vi "Configure.vi"(8 "error in (no error)":errorcluster, 11 "Hardware Refs In":T1={"IP Address"="Simulator", "Handle"=0, "Refresh Time (ms)"=0.0}) -> (0 "error out":errorcluster, 3 "Hardware Refs Out":T1={"IP Address"="Simulator", "Handle"=0, "Refresh Time (ms)"=0.0})   [LabVIEW 2013, in "Capacitive.lvlib"]
uses:
  Capacitive.lvlib
  Hardware Configuration.ctl
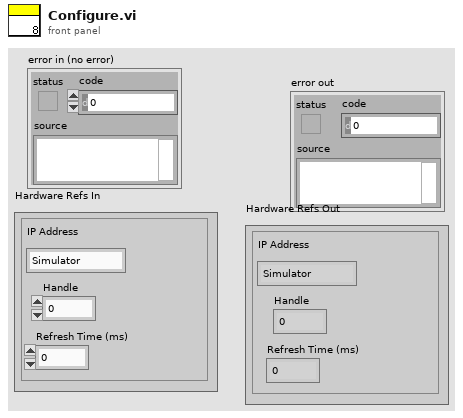
[diagram p1: front panel]
types:
  T1 = typedef "Capacitive.lvlib/Hardware Configuration.ctl" = cluster{"IP Address":string, "Handle":u32, "Refresh Time (ms)":dbl}
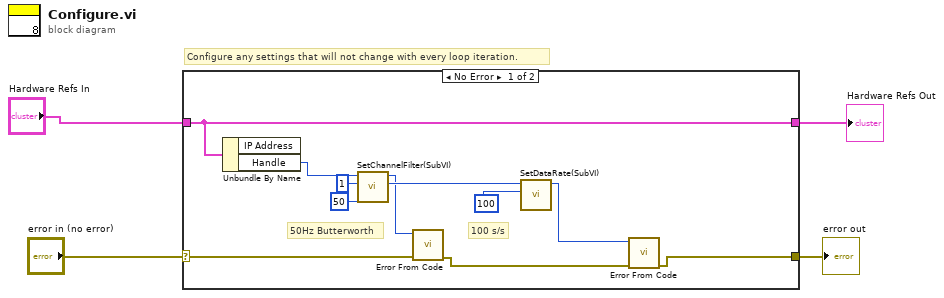
[diagram p0: block diagram]
diagram:
  # "Configure any settings that will not change with every loop iteration."
  n1 = case shown="No Error" "error in (no error)" {
    selector: "error in (no error)" -> [w8 w16]
    tunnel: [w5 w16] -> w3
    tunnel: "Hardware Refs In" -> [w15 w17]
    tunnel: [w15 w17] -> w2
    frame No Error {
      # "100 s/s"
      # "50Hz Butterworth"
      n2 = Unbundle By Name(w15) -> ("Handle"=w14:u32)  [unwired: 1 out]
      n3 = call "SetChannelFilter(SubVI).vi"("FilterNumber"=50, "Channel"=1, "Handle"=w14) -> ("Handle"=w11:u32, "Status"=w9:i32)  [unwired: 4 in, 2 out]
      n4 = call "Error From Code.vi"("error in (no error)"=w8, "ErrorCode"=w9) -> ("error out"=w7:errorcluster)  [unwired: 9 in]
      n5 = call "SetDataRate(SubVI).vi"("DataRate"=100, "Handle"=w11) -> ("Status"=w6:i32)  [unwired: 7 in, 2 out]
      n6 = call "Error From Code.vi"("error in (no error)"=w7, "ErrorCode"=w6) -> ("error out"=w5:errorcluster)  [unwired: 9 in]
    }
    frame Error {
    }
  }
  "error out" <- w3
  "Hardware Refs Out" <- w2
